vi "table_create.vi"(8 "error in (no error)":errorcluster, 10 "table name":string, 11 "toml in":refnum<class "toml.lvclass">) -> (0 "error out":errorcluster, 2 "table created":bool, 3 "toml out":refnum<class "toml.lvclass">)   [LabVIEW 2020, in "toml.lvclass"]
doc: "Will create a new table if a table with the same name doesn't already exist"
uses:
  toml.lvclass
  toml.lvclass/toml.ctl
  Table/Table.lvclass
  Doc/Doc.lvclass
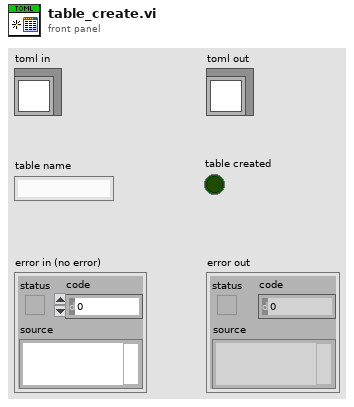
[diagram p1: front panel]
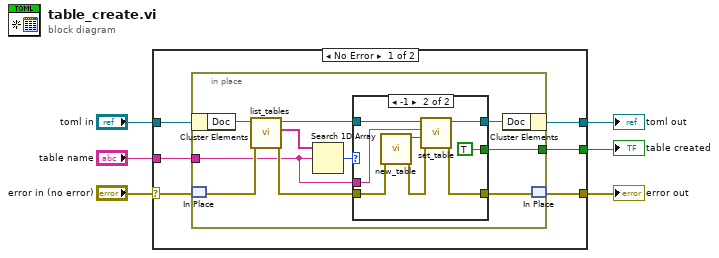
[diagram p0: block diagram]
diagram:
  n1 = case shown="No Error" "error in (no error)" {
    selector: "error in (no error)" -> [w10 w34]
    tunnel: [w9 w34] -> w5
    tunnel: [w11 w33] -> w3
    tunnel: "toml in" -> [w12 w33]
    tunnel: "table name" -> [w8 _]
    tunnel: [w7 _] -> w1
    frame No Error {
      n2 = in-place {
        in-place-border: w8 -> [w13]
        in-place-border: [w16] -> w7
        n3 = in-place-cluster #1(w12) -> ("Doc"=w20:refnum<class "Doc.lvclass">)
        n4 = in-place-match #2(w10) -> (w15:errorcluster)
        n5 = call "list_tables.vi"("error in (no error)"=w15, "Doc in"=w20) -> ("error out"=w14:errorcluster, "table_names"=w18:string[], "Doc out"=w19:refnum<class "Doc.lvclass">)  [unwired: 7 in]
        n6 = Search 1D Array(1D array=w18, element=w13) -> (index of element=w17:i32)  [unwired: 1 in]
        n7 = case shown="-1" w17 {
          tunnel: [w24 w30] -> w22
          tunnel: w14 -> [w23 w29]
          tunnel: [w23 w28] -> w21
          tunnel: w19 -> [w24 w27]
          tunnel: w13 -> [_ w26]
          tunnel: [_ TRUE] -> w16
          frame 0, Default {
          }
          frame -1 {
            n8 = call "new_table.vi"("error in (no error)"=w29) -> ("error out"=w31:errorcluster, "Table out"=w32:refnum<class "Table.lvclass">)  [unwired: 9 in]
            n9 = call "set_table.vi"("error in (no error)"=w31, "Table"=w32, "table_name"=w26, "Doc in"=w27) -> ("error out"=w28:errorcluster, "Doc out"=w30:refnum<class "Doc.lvclass">)  [unwired: 6 in]
          }
        }
        n10 = in-place-cluster #1("Doc"=w22) -> (w11:refnum<class "toml.lvclass">)
        n11 = in-place-match #2(w21) -> (w9:errorcluster)
      }
    }
    frame Error {
    }
  }
  "error out" <- w5
  "toml out" <- w3
  "table created" <- w1
